vi "LogTemerature.vi"(8 "error in (no error)":errorcluster, 11 "Temp_Data":string) -> (0 "error out":errorcluster)   [LabVIEW 2019]
uses:
  <vilib>/Utility/file.llb/Write Delimited Spreadsheet (string).vi
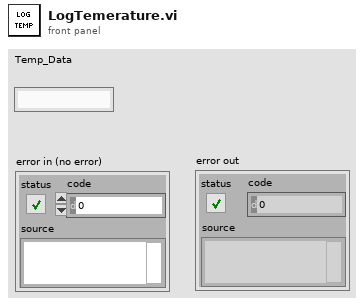
[diagram p1: front panel]
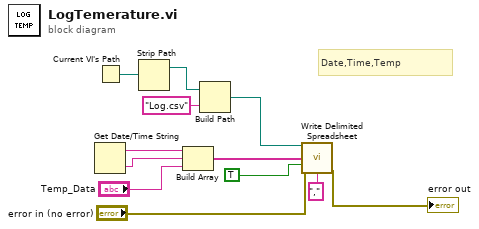
[diagram p0: block diagram]
diagram:
  # "Date,Time,Temp"
  n1 = Get Date/Time String() -> (date string=w11:string, time string=w10:string)  [unwired: 3 in]
  n2 = Current VI's Path() -> (path=w12:path)
  n3 = Strip Path(path=w12) -> (stripped path=w3:path)  [unwired: 1 out]
  n4 = Build Array(w11, w10, "Temp_Data") -> (w8:string[])
  n5 = Build Path(base path=w3, name or relative path="Log.csv") -> (appended path=w1:path)
  n6 = call-poly <vilib>:"Write Delimited Spreadsheet.vi"("file path (dialog if empty)"=w1, "1D data"=w8, "append to file? (new file:F)"=TRUE, "error in (no error)"="error in (no error)", "delimiter (\\t)"="," ("delimiter (\\t)")) -> ("error out"=→"error out":errorcluster)  [unwired: 9 in, 1 out]
